vi "get subpanel value.vi"(8 "error in (no error)":errorcluster, 11 "JSON string":string) -> (0 "error out":errorcluster, 3 "value":string)   [LabVIEW 2020, in "ui-testing.lvlib"]
doc: "copyright: Thomas Zilliox©"
uses:
  ui-testing.lvlib
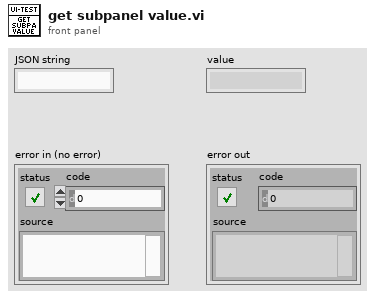
[diagram p1: front panel]
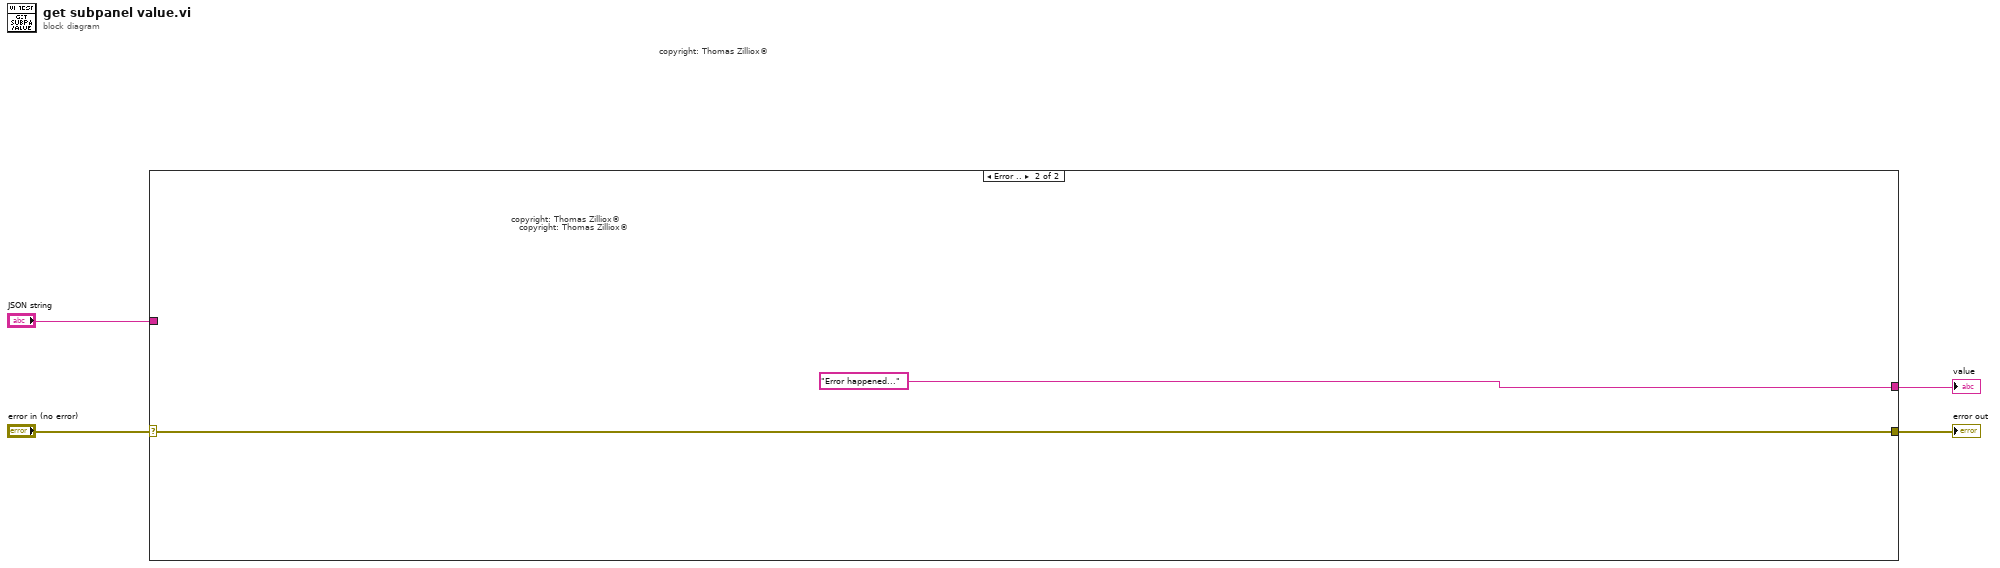
[diagram p0: block diagram]
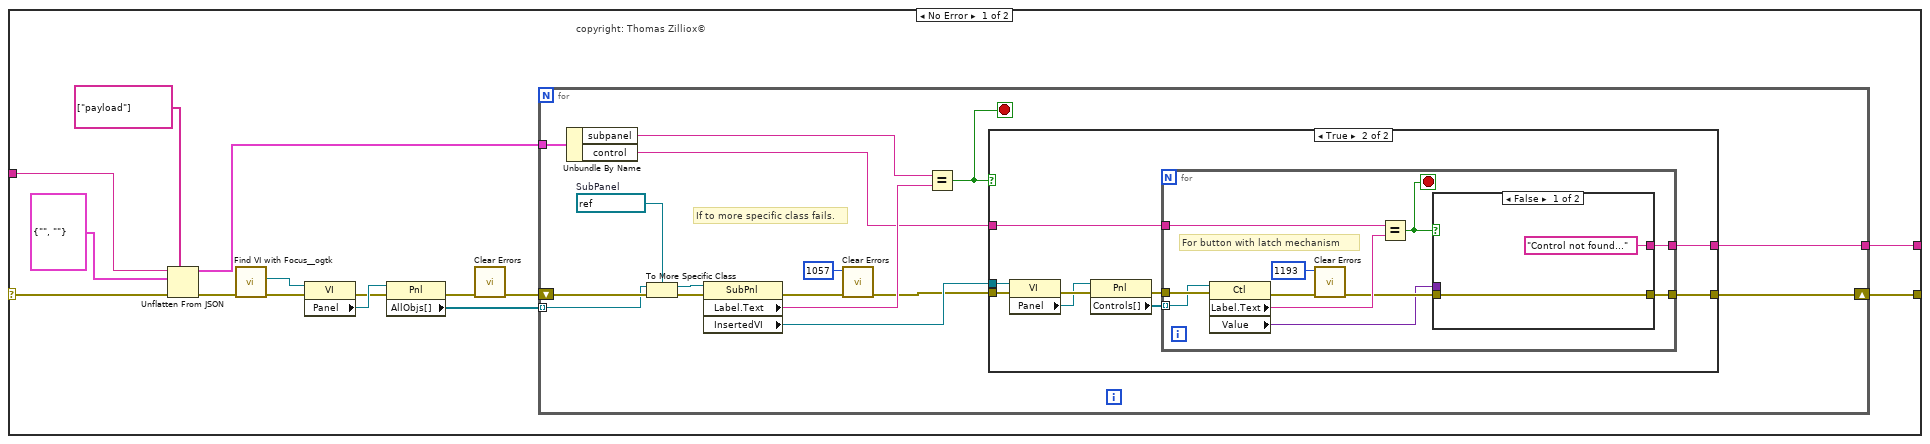
[diagram p2: hidden frame]
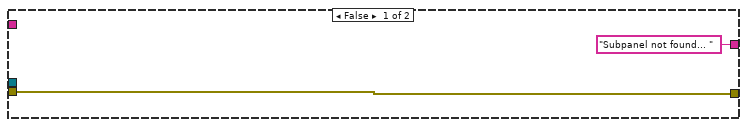
[diagram p3: hidden frame]
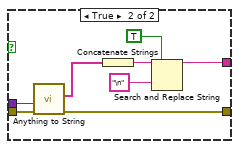
[diagram p4: hidden frame]
diagram:
  # "copyright: Thomas Zilliox©"
  n1 = case shown="Error .." "error in (no error)" {
    selector: "error in (no error)" -> [w8 w69]
    tunnel: "JSON string" -> [w12 _]
    tunnel: [w9 w69] -> w3
    tunnel: [w5 "Error happened..."] -> w1
    frame No Error {
      # "copyright: Thomas Zilliox©"
      n2 = Unflatten From JSON(path=string[] ["payload"], JSON string=w12, type and defaults=cluster{"subpanel":string, "control":string} {"subpanel"="", "control"=""}, error in (no error)=w8) -> (value=w6:cluster{"subpanel":string, "control":string}, error out=w13:errorcluster)  [unwired: 3 in]
      n3 = call <userlib>:"Find VI with Focus__ogtk.vi"("error in"=w13) -> ("error out"=w18:errorcluster, "VI with Focus"=w17:refnum<vi>)  [unwired: 6 in, 3 out]
      n4 = property class="VI"(reference=w17, error in=w18) -> (error out=w14:errorcluster, "Panel"=w16:refnum<vi>)  [unwired: 1 out]
      n5 = property class="Pnl"(reference=w16, error in=w14) -> (error out=w11:errorcluster, "AllObjs[]"=w15:refnum<vi>[])  [unwired: 1 out]
      n6 = call <vilib>:"Clear Errors.vi"("error in (no error)"=w11) -> ("error out"=w10:errorcluster)  [unwired: 5 in, 1 out]
      n7 = for {
        tunnel: w15 -> [w31] mode=indexing
        shift-right: [w23] -> w9
        shift-left: w10 -> [w32]
        tunnel: w6 -> [w30]
        tunnel: [w24] -> w5
        stop <- w25 stop-if-true
        w35 = refnum<vi> refnum  # SubPanel
        # "If to more specific class fails."
        n8 = Unbundle By Name(w30) -> ("subpanel"=w29:string, "control"=w26:string)
        n9 = To More Specific Class(target class=w35, reference=w31, error in=w32) -> (specific class reference=w34:refnum<vi>, error out=w33:errorcluster)
        n10 = property class="SubPnl"(reference=w34, error in=w33) -> (error out=w22:errorcluster, "Label.Text"=w28:string, "InsertedVI"=w27:refnum<vi>)  [unwired: 1 out]
        n11 = call <vilib>:"Clear Errors.vi"("error in (no error)"=w22, "specific error code to clear (0: all)"=1057) -> ("error out"=w21:errorcluster)  [unwired: 4 in, 1 out]
        n12 = Equal?(x=w29, y=w28) -> (x = y?=w25:bool)
        n13 = case shown="True" w25 {
          tunnel: [w37 w46] -> w23
          tunnel: w27 -> [_ w43]
          tunnel: w21 -> [w37 w42]
          tunnel: w26 -> [_ w39]
          tunnel: ["Subpanel not found... " ("result string") w38] -> w24
          frame False {
          }
          frame True {
            n14 = property class="VI"(reference=w43, error in=w42) -> (error out=w45:errorcluster, "Panel"=w44:refnum<vi>)  [unwired: 1 out]
            n15 = property class="Pnl"(reference=w44, error in=w45) -> (error out=w41:errorcluster, "Controls[]"=w40:refnum<vi>[])  [unwired: 1 out]
            n16 = for {
              tunnel: [w49] -> w46
              tunnel: w41 -> [w55]
              tunnel: w40 -> [w54] mode=indexing
              tunnel: w39 -> [w53]
              tunnel: [w48] -> w38
              stop <- w47 stop-if-true
              # "For button with latch mechanism"
              n17 = property class="Ctl"(reference=w54, error in=w55) -> (error out=w57:errorcluster, "Label.Text"=w52:string, "Value"=w50:variant)  [unwired: 1 out]
              n18 = call <vilib>:"Clear Errors.vi"("error in (no error)"=w57, "specific error code to clear (0: all)"=1193) -> ("error out"=w51:errorcluster)  [unwired: 4 in, 1 out]
              n19 = Equal?(x=w53, y=w52) -> (x = y?=w47:bool)
              n20 = case shown="False" w47 {
                tunnel: w51 -> [w59 w67]
                tunnel: w50 -> [_ w66]
                tunnel: [w59 w65] -> w49
                tunnel: ["Control not found..." ("result string") w60] -> w48
                frame False {
                }
                frame True {
                  n21 = call <userlib>:"Anything to String.vi"("Error In"=w67, "Anything"=w66) -> ("Error Out"=w65:errorcluster, "Strings[]"=w61:string[])  [unwired: 7 in, 1 out]
                  n22 = Concatenate Strings(w61) -> (w64:string)
                  n23 = Search and Replace String(replace all?=TRUE ("replace all? (F)"), input string=w64, search string="\n") -> (result string=w60:string)  [unwired: 5 in, 3 out]
                }
              }
            }
          }
        }
      }
    }
    frame Error {
      # "copyright: Thomas Zilliox©"
      # "copyright: Thomas Zilliox©"
    }
  }
  "error out" <- w3
  "value" <- w1
